vi "InnerCallbackOnWriteTree.vi"(8 "error in":errorcluster, 10 "node (for type)":refnum<class "E2E Tag Exchange editor node.lvclass">, 11 "node reference":refnum<data-value>) -> (0 "error out":errorcluster)   [LabVIEW 2015, in "E2E Tag Exchange editor node.lvclass"]
doc: "Copyright 2015 National Instruments Corporation\n\nLicensed under the Apache License, Version 2.0 (the \"License\"); you may not use this file except in compliance with the License. You may obtain a copy of the License at http://www.apache.org/licenses/LICENSE-2.0\nUnless required by applicable law or agreed to in writing, software distributed under the License is distributed on an \"AS IS\" BASIS, WITHOUT WARRANTIES OR CONDITIONS OF ANY KIND, either express or implied. See the License for the specific language governing permissions and limitations under the License."
uses:
  E2E Tag Exchange editor node.lvclass
  <vilib>/NI/Configuration Framework/Node/NISE_CEF_Node.lvclass
  Node LUT/Command.ctl
  <vilib>/NI/DCAF/Tag Editor Core/Configuration Editor/Classes/Module editor node/module editor node.lvclass
  Node LUT/Node LUT.lvlib
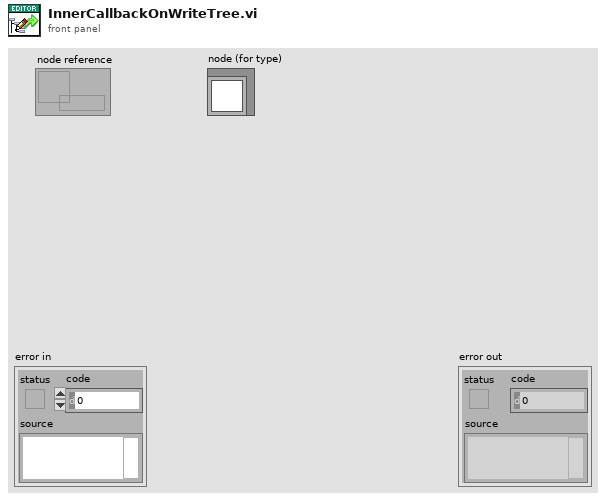
[diagram p1: front panel]
types:
  T1 = typedef "Node LUT.lvlib/Command.ctl" = enum16{"Initialize", "Add Node", "Remove Node", "Node Ref from UID", "List Nodes"}
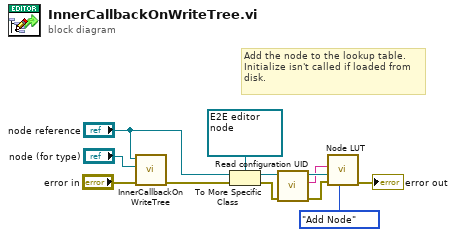
[diagram p0: block diagram]
diagram:
  # "Add the node to the lookup table.\nInitialize isn't called if loaded from\ndisk."
  n1 = call-parent "InnerCallbackOnWriteTree.vi"("error in"="error in", "node (for type)"="node (for type)", "node reference"="node reference") -> ("error out"=w3:errorcluster)  [unwired: 8 in]
  n2 = To More Specific Class(target class=refnum<data-value> refnum, reference="node reference", error in=w3) -> (specific class reference=w9:refnum<data-value>, error out=w5:errorcluster)
  n3 = call "Read configuration UID.vi"("error in (no error)"=w5, "E2E editor node in"=w9) -> ("error out"=w7:errorcluster, "Module UID"=w6:string, "E2E editor node out"=w10:refnum<data-value>)  [unwired: 7 in]
  n4 = call "Node LUT.vi"("Command"=Command."Add Node", "error in"=w7, "node ref"=w10, "UID"=w6) -> ("error out"=→"error out":errorcluster)  [unwired: 4 in, 3 out]
